vi "User & System Details.vi"(8 "error in (no error)":errorcluster) -> (0 "error out":errorcluster, 2 "Boolean":bool, 5 "User Name 2":string caption="שם משתמש", 7 "מספר סידורי 2":string caption="מספר סידורי")   [LabVIEW 2014]
uses:
  <vilib>/Utility/file.llb/Read From Spreadsheet File (string).vi
  <vilib>/Utility/file.llb/Write To Spreadsheet File (string).vi
panel:
  in  "Cancel Button":bool
  in  "Next Button":bool
  in  "User Name":string caption="שם משתמש"
  in  "מספר סידורי":string
  out "Msg":string
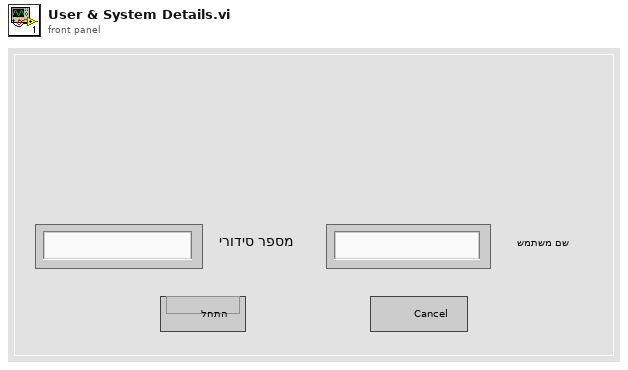
[diagram p1: front panel]
types:
  T1 = enum32{"Invalid", "Standard", "Closed", "Hidden", "Minimized", "Maximized"}
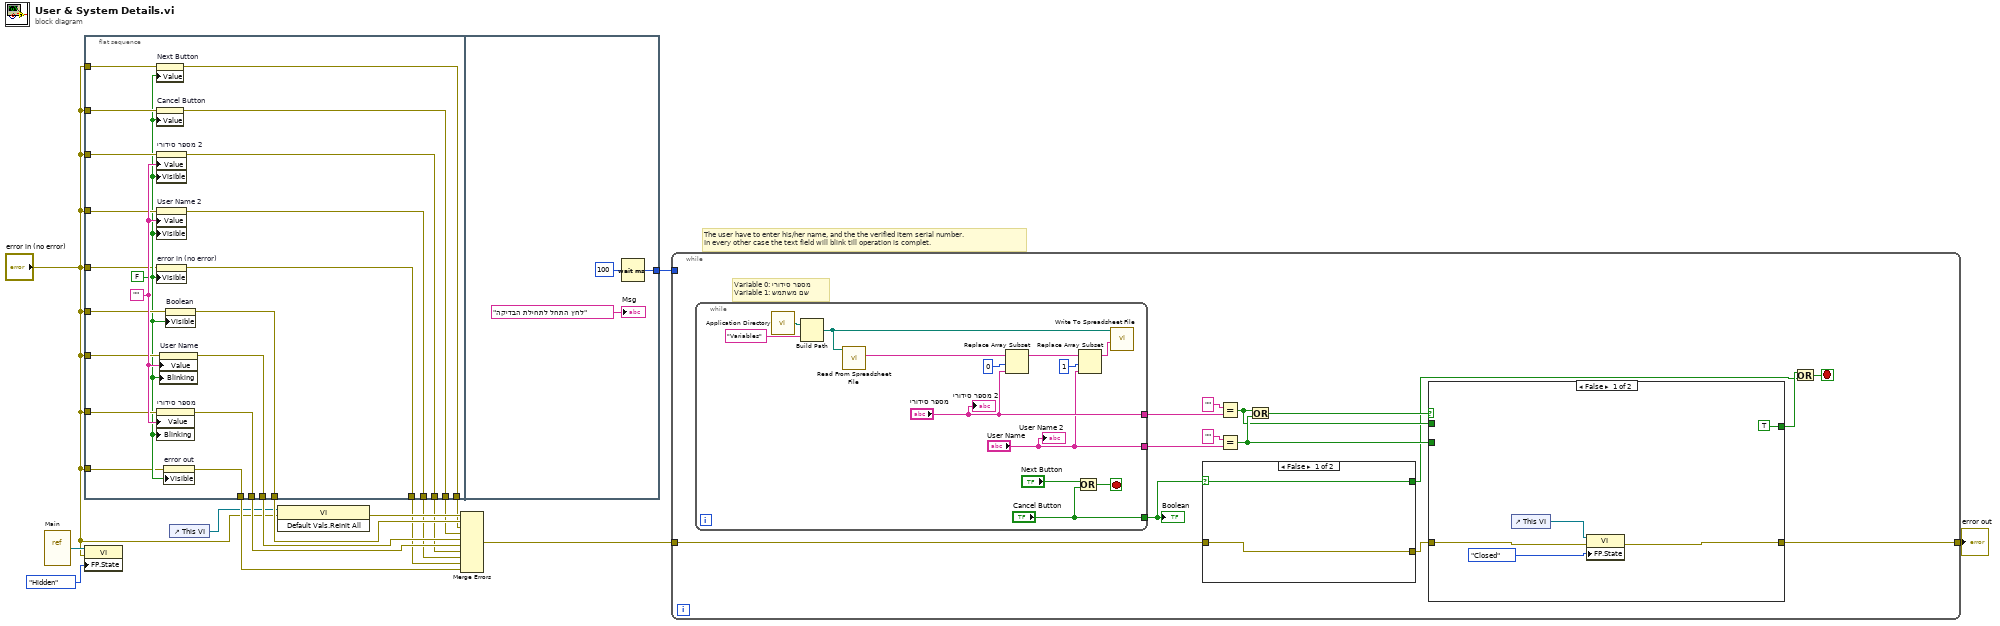
[diagram p0: block diagram]
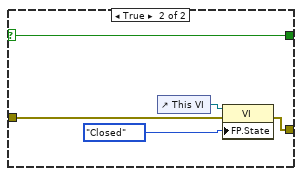
[diagram p2: hidden frame]
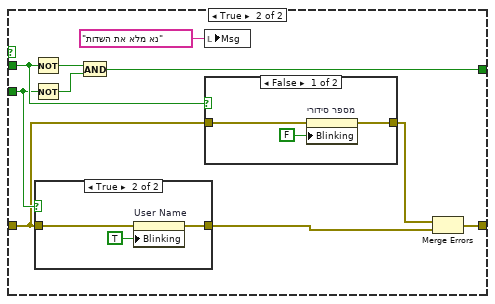
[diagram p3: hidden frame]
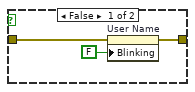
[diagram p4: hidden frame]
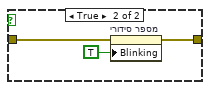
[diagram p5: hidden frame]
diagram:
  # "The user have to enter his/her name, and the the verified item serial number.\nIn every other case the text field will blink till operation is complet."
  n1 = vi-ref "Main.vi"() -> (w4:refnum<vi>)
  n2 = flat-sequence {
    tunnel: "error in (no error)" -> [w36]
    tunnel: "error in (no error)" -> [w35]
    tunnel: "error in (no error)" -> [w34]
    tunnel: "error in (no error)" -> [w33]
    tunnel: "error in (no error)" -> [w32]
    tunnel: "error in (no error)" -> [w31]
    tunnel: "error in (no error)" -> [w30]
    tunnel: [w29] -> w15
    tunnel: [w28] -> w14
    tunnel: [w27] -> w13
    tunnel: [w26] -> w12
    tunnel: [w25] -> w11
    tunnel: [w24] -> w10
    tunnel: [w23] -> w9
    tunnel: "error in (no error)" -> [w21]
    tunnel: "error in (no error)" -> [w20]
    tunnel: [w19] -> w7
    tunnel: [w18] -> w6
    tunnel: [w39] -> w17
    frame #0 {
      w37 = ""
      w22 = FALSE
      n3 = property on="Next Button" class="Bool (strict)"(error in=w35, "Value"=w22) -> (error out=w28:errorcluster)  [unwired: 1 in, 1 out]
      n4 = property on="Cancel Button" class="Bool (strict)"(error in=w34, "Value"=w22) -> (error out=w27:errorcluster)  [unwired: 1 in, 1 out]
      n5 = property on="מספר סידורי 2" class="Str"(error in=w31, "Value"=w37, "Visible"=w22) -> (error out=w24:errorcluster)  [unwired: 1 in, 1 out]
      n6 = property on="User Name 2" class="Str"(error in=w30, "Value"=w37, "Visible"=w22) -> (error out=w23:errorcluster)  [unwired: 1 in, 1 out]
      n7 = property on="error in (no error)" class="Clust (strict)"(error in=w20, "Visible"=w22) -> (error out=w19:errorcluster)  [unwired: 1 in, 1 out]
      n8 = property on="מספר סידורי" class="Str"(error in=w32, "Value"=w37, "Blinking"=w22) -> (error out=w25:errorcluster)  [unwired: 1 in, 1 out]
      n9 = property on="User Name" class="Str"(error in=w33, "Value"=w37, "Blinking"=w22) -> (error out=w26:errorcluster)  [unwired: 1 in, 1 out]
      n10 = property on="error out" class="Clust (strict)"(error in=w21, "Visible"=w22) -> (error out=w18:errorcluster)  [unwired: 1 in, 1 out]
      n11 = property on="Boolean" class="Bool (strict)"(error in=w36, "Visible"=w22) -> (error out=w29:errorcluster)  [unwired: 1 in, 1 out]
    }
    frame #1 {
      n12 = Wait (ms)(milliseconds to wait=u32 100) -> (millisecond timer value=w39:u32)
      "Msg" <- "לחץ התחל לתחילת הבדיקה" ("mainMsg")
    }
  }
  n13 = property class="VI"(reference=w4, error in="error in (no error)", "FP.State"=T1."Hidden" ("Front Panel Window:State")) -> ()  [unwired: 2 out]
  n14 = control-ref of="This VI"() -> (w5:refnum<vi>)
  n15 = invoke class="VI" method="Default Vals.Reinit All"(reference=w5, error in="error in (no error)") -> (error out=w16:errorcluster)  [unwired: 1 in, 2 out]
  n16 = Merge Errors(w16, w15, w14, w13, w12, w11, w10, w9, w7, w6) -> (w8:errorcluster)
  n17 = while {
    tunnel: w17 -> [_]
    tunnel: w8 -> [w44]
    tunnel: [w45] -> w1
    stop <- w46 stop-if-true
    # "Variable 0: מספר סידורי\nVariable 1: שם משתמש"
    n18 = while {
      tunnel: ["מספר סידורי"] -> w49
      tunnel: ["User Name"] -> w48
      tunnel: ["Cancel Button"] -> w42
      stop <- w90 stop-if-true
      n19 = call <vilib>:"Application Directory.vi"() -> ("Application Directory"=w100:path)
      n20 = Build Path(base path=w100, name or relative path="Variables") -> (appended path=w98:path)
      n21 = call-poly <vilib>:"Read From Spreadsheet File.vi"("file path (dialog if empty)"=w98) -> ("first row"=w99:string[])  [unwired: 6 in, 4 out]
      n22 = Replace Array Subset(array=w99, new element="מספר סידורי", index=0) -> (w94:string[])
      n23 = Or(x="Next Button", y="Cancel Button") -> (x .or. y?=w90:bool)
      n24 = Replace Array Subset(array=w94, new element="User Name", index=1) -> (w95:string[])
      n25 = call-poly <vilib>:"Write To Spreadsheet File.vi"("1D data"=w95, "file path (dialog if empty)"=w98) -> ()  [unwired: 6 in, 1 out]
      "מספר סידורי 2" <- "מספר סידורי"
      "User Name 2" <- "User Name"
    }
    "Boolean" <- w42
    n26 = case shown="False" w42 {
      selector: w42 -> [w56 w61]
      tunnel: [w56 w61] -> w41
      tunnel: w44 -> [w55 w58]
      tunnel: [w55 w57] -> w43
      frame False {
      }
      frame True {
        n27 = control-ref of="This VI"() -> (w59:refnum<vi>)
        n28 = property class="VI"(reference=w59, error in=w58, "FP.State"=T1."Closed" ("Front Panel Window:State")) -> (error out=w57:errorcluster)  [unwired: 1 out]
      }
    }
    n29 = Equal?(x="", y=w49) -> (x = y?=w52:bool)
    n30 = Equal?(x="", y=w48) -> (x = y?=w53:bool)
    n31 = Or(x=w52, y=w53) -> (x .or. y?=w54:bool)
    n32 = case shown="False" w54 {
      tunnel: w52 -> [_ w76]
      tunnel: w53 -> [_ w75]
      tunnel: [TRUE w71] -> w47
      tunnel: w43 -> [w66 w70]
      tunnel: [w65 w69] -> w45
      frame False {
        n33 = control-ref of="This VI"() -> (w63:refnum<vi>)
        n34 = property class="VI"(reference=w63, error in=w66, "FP.State"=T1."Closed" ("Front Panel Window:State")) -> (error out=w65:errorcluster)  [unwired: 1 out]
      }
      frame True {
        n35 = Not(x=w76) -> (.not. x?=w74:bool)
        n36 = Not(x=w75) -> (.not. x?=w73:bool)
        n37 = case shown="True" w75 {
          tunnel: w70 -> [w78 w81]
          tunnel: [w77 w80] -> w67
          frame False {
            n38 = property on="User Name" class="Str"(error in=w78, "Blinking"=FALSE) -> (error out=w77:errorcluster)  [unwired: 1 in, 1 out]
          }
          frame True {
            n39 = property on="User Name" class="Str"(error in=w81, "Blinking"=TRUE) -> (error out=w80:errorcluster)  [unwired: 1 in, 1 out]
          }
        }
        n40 = And(x=w74, y=w73) -> (x .and. y?=w71:bool)
        n41 = local write "Msg"("נא מלא את השדות" ("Msg")) -> ()
        n42 = case shown="False" w76 {
          tunnel: w70 -> [w84 w87]
          tunnel: [w83 w86] -> w68
          frame False {
            n43 = property on="מספר סידורי" class="Str"(error in=w84, "Blinking"=FALSE) -> (error out=w83:errorcluster)  [unwired: 1 in, 1 out]
          }
          frame True {
            n44 = property on="מספר סידורי" class="Str"(error in=w87, "Blinking"=TRUE) -> (error out=w86:errorcluster)  [unwired: 1 in, 1 out]
          }
        }
        n45 = Merge Errors(w68, w67) -> (w69:errorcluster)
      }
    }
    n46 = Or(x=w47, y=w41) -> (x .or. y?=w46:bool)
  }
  "error out" <- w1
